vi "Sim Read AI DAQ Data.vi"(0 "DAQ Node Dict DVR":T2, 1 "IP_RawDataQ":T1, 2 "TDMS_RawDataQ":T1, 3 "AI TaskName":string, 5 "DAQ Data Dict DVR":T2, 7 "AI IONames":string[](array[string]), 9 "SimAI Ranges":T3, 11 "error in":errorcluster) -> (4 "DAQ Node Dict DVR out":T2, 6 "DAQ Data Dict DVR out":T2, 15 "error out":errorcluster)   [LabVIEW 2017, in "DAQ.lvclass"]
doc: "Developed by Kevin Thompson\nkevin@thompsonengineering.net\n\nCopyright 2018-2020\nThompson Engineering, LLC\nAI scan timestamp is stored with IOName \"AIScanTS\" in DAQ Data Dict.\nAI scan array is stored with IOName \"AIScanArray\" in DAQ Data Dict.\n[AI IONames] input is obtained from AI IOName enum TD"
uses:
  DAQ.lvclass
  TD SimAI Ranges--cluster.ctl
  <vilib>/TELLC/Dynamic CVT API/TD Dynamic CVT DVR--ref.ctl
  Support/DataQueues/DataTypes/Analog DataSet MultiRow & ChanNames--QRef.ctl
  Support/DataQueues/DataTypes/Analog DataSet MultiRow & ChanNames--cluster.ctl
  Support/DataQueues/DataQueues.lvclass
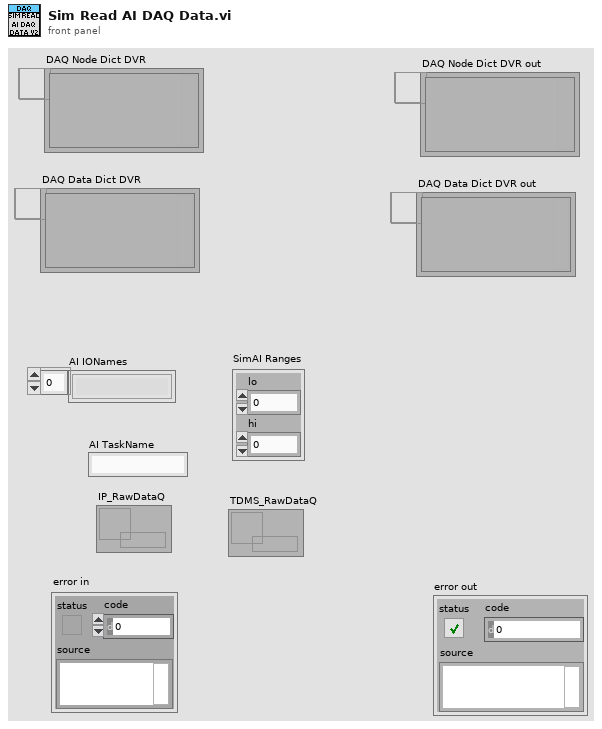
[diagram p1: front panel]
types:
  T1 = typedef "DataQueues.lvclass/Analog DataSet MultiRow & ChanNames--QRef.ctl" = refnum<queue>
  T2 = typedef "TD Dynamic CVT DVR--ref.ctl" = refnum<data-value>
  T3 = typedef "DAQ.lvclass/TD SimAI Ranges--cluster.ctl" = cluster{"lo":dbl, "hi":dbl}
  T4 = typedef "DataQueues.lvclass/Analog DataSet MultiRow & ChanNames--cluster.ctl" = cluster{"TimeStamp_(s)":dbl, "data":dbl[][], "ChanNames":string[]}
  T5 = typedef "DAQ.lvclass/TD local raw AI Data--cluster.ctl" = cluster{"TimeStamp_(s)":dbl, "data":dbl[][]}
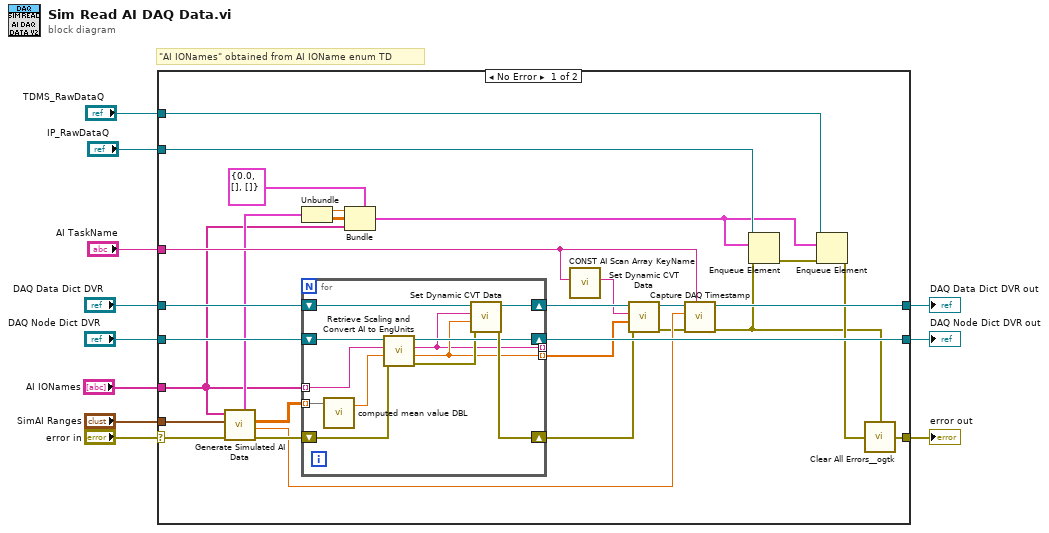
[diagram p0: block diagram]
diagram:
  # "\"AI IONames\" obtained from AI IOName enum TD"
  n1 = case shown="No Error" "error in" {
    selector: "error in" -> [w35 w53]
    tunnel: "SimAI Ranges" -> [w31 _]
    tunnel: "DAQ Data Dict DVR" -> [w39 w54]
    tunnel: [w38 w54] -> w9
    tunnel: [w19 w53] -> w8
    tunnel: "DAQ Node Dict DVR" -> [w37 w52]
    tunnel: [w36 w52] -> w5
    tunnel: "AI IONames" -> [w13 _]
    tunnel: "AI TaskName" -> [w25 _]
    tunnel: "IP_RawDataQ" -> [w23 _]
    tunnel: "TDMS_RawDataQ" -> [w20 _]
    frame No Error {
      n2 = call "Generate Simulated AI Data.vi"("error in"=w35, "SimRange"=w31, "IONames[]"=w13) -> ("error out"=w33:errorcluster, "timestamp"=w32:dbl, "data"=w34:dbl[][], "Q element"=w14:T5)  [unwired: 5 in]
      n3 = Unbundle(w14) -> ("TimeStamp_(s)"=w15:dbl, "data"=w16:dbl[][])
      n4 = for {
        tunnel: w34 -> [w51] mode=indexing
        tunnel: w13 -> [w43] mode=indexing
        shift-right: [w49] -> w27
        shift-left: w39 -> [w50]
        shift-right: [w48] -> w30
        shift-left: w33 -> [w46]
        shift-right: [w45] -> w36
        shift-left: w37 -> [w47]
        tunnel: [w41] -> w28 mode=indexing
        tunnel: [w40] -> _ mode=indexing
        n5 = call <vilib>:"computed mean value DBL.vi"("Array in"=w51) -> ("MeanValue"=w44:dbl)  [unwired: 1 out]
        n6 = call "Retrieve Scaling and Convert AI to EngUnits.vi"("error in (no error)"=w46, "RawValue in"=w44, "IOName"=w43, "DAQ Node Dict DVR"=w47) -> ("error out"=w42:errorcluster, "Engineering Units Out"=w41:dbl, "IOName out"=w40:string, "DAQ Node Dict DVR out"=w45:T2)  [unwired: 4 in]
        n7 = call <vilib>:"Set Dynamic CVT Data.vi"("error in (no error)"=w42, "value"=w41, "DataName"=w40, "dCVT DVR"=w50) -> ("error out"=w48:errorcluster, "dCVT DVR out"=w49:T2)  [unwired: 5 in, 1 out]
      }
      n8 = Bundle(cluster=T4 {"TimeStamp_(s)"=0.0, "data"=[], "ChanNames"=[]} ("Analog DataSet MultiRow & ChanNames"), "TimeStamp_(s)"=w15, "data"=w16, "ChanNames"=w13) -> (w12:T4)
      n9 = call "CONST AI Scan Array KeyName.vi"("AI TaskName"=w25) -> ("AI ScanArray (KeyName)"=w24:string)  [unwired: 10 in]
      n10 = call <vilib>:"Set Dynamic CVT Data.vi"("error in (no error)"=w30, "value"=w28, "DataName"=w24, "dCVT DVR"=w27) -> ("error out"=w29:errorcluster, "dCVT DVR out"=w26:T2)  [unwired: 5 in, 1 out]
      n11 = call "Capture DAQ Timestamp.vi"("DaqData dCVT"=w26, "timestamp in"=w32, "error in (no error)"=w29, "AI TaskName"=w25) -> ("DaqData dCVT out"=w38:T2, "error out"=w18:errorcluster)  [unwired: 4 in, 1 out]
      n12 = Enqueue Element(queue=w23, element=w12, error in (no error)=w18) -> (error out=w22:errorcluster)  [unwired: 1 in, 2 out]
      n13 = Enqueue Element(queue=w20, element=w12, error in (no error)=w22) -> (error out=w21:errorcluster)  [unwired: 1 in, 2 out]
      n14 = call <userlib>:"Clear All Errors__ogtk.vi"("Upsteam Error (optional)"=w18, "Error In"=w21) -> ("Error Out"=w19:errorcluster)  [unwired: 2 in]
    }
    frame Error {
    }
  }
  "DAQ Data Dict DVR out" <- w9
  "error out" <- w8
  "DAQ Node Dict DVR out" <- w5
